vi "MidbrainArbiter.vi"(0 "ForebrainInput":dbl[](array[numeric]), 5 "ObstacleAvoid":dbl[](array[numeric]), 7 "Wall Follow":dbl[](array[numeric]), 9 "Lane Follow":dbl[](array[numeric]), 11 "Wall Avoid":dbl[](array[numeric])) -> (8 "Act Command":cluster{"Velocity":dbl, "Direction":dbl})   [LabVIEW 2010]
doc: "This VI arbitrates the one command input form the Forebrain, and a set of inputs from the Limbic and Cerrebellum THINK processes and conducts a voting poll arbitor with input from each to determine the one output command.\n\nInputs: 90 cell arrays of weighted direction commands \n\nOutput: Cluster of desried velocity and direction"
panel:
  out "Waveform Graph":dbl[][](graph)
  # "This subVI takes the three\nACT commands; one from the forebrain \nand three from the Midbrain and\naverages them"
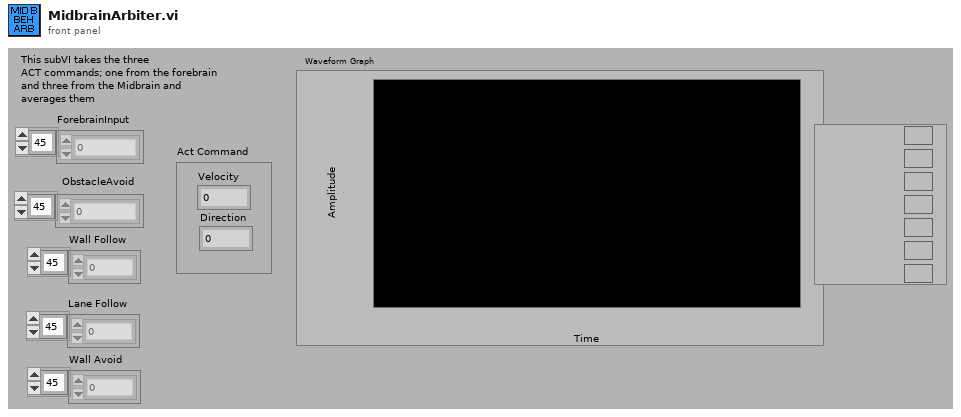
[diagram p1: front panel]
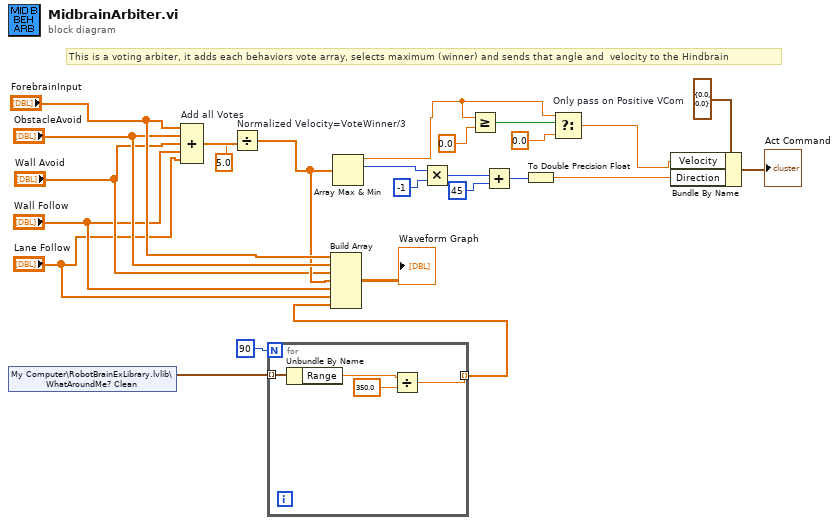
[diagram p0: block diagram]
diagram:
  # "This is a voting arbiter, it adds each behaviors vote array, selects maximum (winner) and sends that angle and  velocity to the Hindbrain"
  n1 = shared-variable "My Computer\\RobotBrainExLibrary.lvlib\\WhatAroundMe? Clean"() -> (w4:cluster{"T":dbl, "Range":dbl, "Bearing":dbl}[])  [unwired: 1 in, 1 out]
  n2 = Compound Arithmetic op=ADD "Add all Votes"("ForebrainInput", "ObstacleAvoid", "Wall Avoid", "Wall Follow", "Lane Follow") -> (w14:dbl[])
  n3 = Divide "Normalized Velocity=VoteWinner/3"(x=w14, y=5.0) -> (x/y=w7:dbl[])
  n4 = for {
    N: 90 -> [_]
    tunnel: w4 -> [w29] mode=indexing
    tunnel: [w27] -> w2 mode=indexing
    n5 = Unbundle By Name(w29) -> ("Range"=w28:dbl)
    n6 = Divide(x=w28, y=350.0) -> (x/y=w27:dbl)
  }
  n7 = Build Array "Build Array"("ForebrainInput", "ObstacleAvoid", "Wall Avoid", w7, "Wall Follow", "Lane Follow", w2) -> (→"Waveform Graph":dbl[][])
  n8 = Array Max & Min(array=w7) -> (max value=w10:dbl, max index (indices)=w23:i32)  [unwired: 2 out]
  n9 = Multiply(x=w23, y=-1) -> (x*y=w21:i32)
  n10 = Greater Or Equal?(x=w10, y=0.0) -> (x >= y?=w11:bool)
  n11 = Add(x=w21, y=45) -> (x+y=w19:i32)
  n12 = To Double Precision Float(number=w19) -> (double precision float=w18:dbl)
  n13 = Select "Only pass on Positive VCom"(t=w10, s=w11, f=0.0) -> (s? t:f=w8:dbl)
  n14 = Bundle By Name(cluster=cluster{"Velocity":dbl, "Direction":dbl} {"Velocity"=0.0, "Direction"=0.0} ("Act Command"), "Velocity"=w8, "Direction"=w18) -> (→"Act Command":cluster{"Velocity":dbl, "Direction":dbl})
